vi "Get Channel Resistance.vi"(8 "error in (no error)":errorcluster, 10 "Params":variant, 11 "Programmable Resistor in":refnum<class "Programmable Resistor.lvclass">) -> (0 "error out":errorcluster, 2 "Value":variant, 3 "Programmable Resistor out":refnum<class "Programmable Resistor.lvclass">)   [LabVIEW 2020, in "Instrument.lvlib" / "Programmable Resistor.lvclass"]
uses:
  Programmable Resistor.lvclass
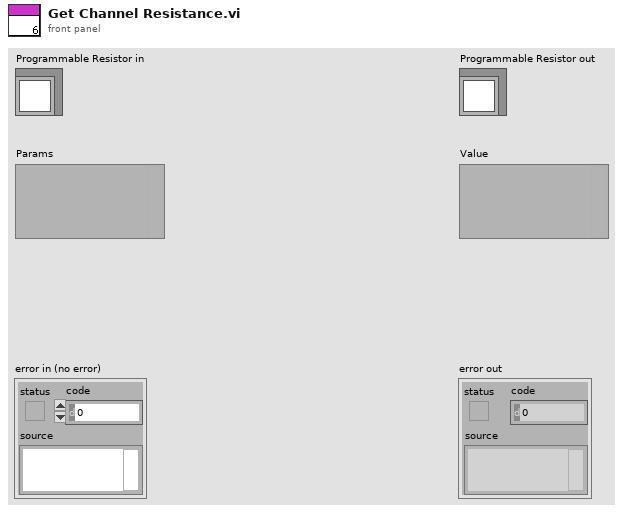
[diagram p1: front panel]
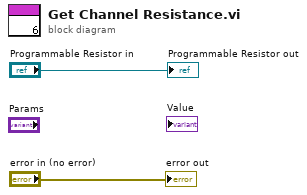
[diagram p0: block diagram]
diagram:
  "error out" <- "error in (no error)"
  "Programmable Resistor out" <- "Programmable Resistor in"
